vi "ConvertCountsToUnits.vi"(8 "error in (no error)":errorcluster, 10 "Coordinates.Counts":T1, 11 "XYStage in":refnum<class "XYStage.lvclass">) -> (0 "error out":errorcluster, 2 "Coordinates.Units":T2, 3 "XYStage out":refnum<class "XYStage.lvclass">)   [LabVIEW 2019, in "XYStage.lvclass"]
uses:
  XYStage.lvclass
  Typedefs/Coordinates.Units--Cluster.ctl
  Typedefs/Coordinates.Counts--Cluster.ctl
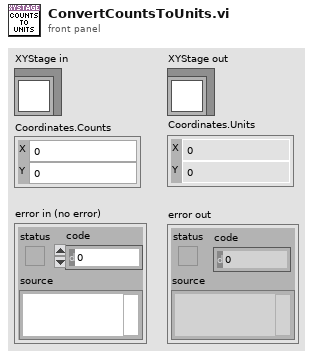
[diagram p1: front panel]
types:
  T1 = typedef "XYStage.lvclass/Coordinates.Counts--Cluster.ctl" = cluster{"X":i32, "Y":i32}
  T2 = typedef "XYStage.lvclass/Coordinates.Units--Cluster.ctl" = cluster{"X":dbl, "Y":dbl}
  T3 = typedef "XYStage.lvclass/Configuration--Cluster.ctl" = cluster{"Serial Number":string, "X Axis":string, "Y Axis":string, "Real-World Units":string, "Counts per Unit":u32}
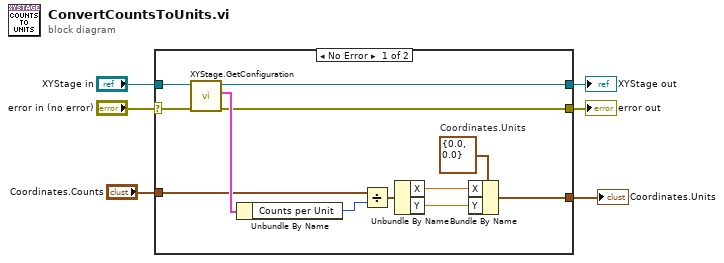
[diagram p0: block diagram]
diagram:
  n1 = case shown="No Error" "error in (no error)" {
    selector: "error in (no error)" -> [w17 w20]
    tunnel: [w14 w20] -> w5
    tunnel: [w15 w19] -> w3
    tunnel: "XYStage in" -> [w18 w19]
    tunnel: "Coordinates.Counts" -> [w13 _]
    tunnel: [w7 _] -> w1
    frame No Error {
      w10 = T2 {"X"=0.0, "Y"=0.0}  # Coordinates.Units
      n2 = call "XYStage.GetConfiguration.vi"("error in (no error)"=w17, "XYStage"=w18) -> ("error out"=w14:errorcluster, "Configuration"=w16:T3, "XYStage out"=w15:refnum<class "XYStage.lvclass">)  [unwired: 7 in]
      n3 = Unbundle By Name(w16) -> ("Counts per Unit"=w12:u32)
      n4 = Divide(x=w13, y=w12) -> (x/y=w11:cluster{"X":dbl, "Y":dbl})
      n5 = Unbundle By Name(w11) -> ("X"=w9:dbl, "Y"=w8:dbl)
      n6 = Bundle By Name(cluster=w10, "X"=w9, "Y"=w8) -> (w7:T2)
    }
    frame Error {
    }
  }
  "error out" <- w5
  "XYStage out" <- w3
  "Coordinates.Units" <- w1
